vi "Add Command.vi"(8 "error in (no error)":errorcluster, 9 "Index":i32=-1 min=-1 step=1, 10 "Write Command":refnum<class "WriteCommand.lvclass">, 11 "Command Director in":refnum<class "CommandDirector.lvclass">) -> (0 "error out":errorcluster, 3 "Command Director out":refnum<class "CommandDirector.lvclass">)   [LabVIEW 2023, in "HAF.lvlib" / "CommandDirector.lvclass"]
doc: "Adds a Command to a given position in the current collection. If Index is not provided, then adds at the end. Collection is zero indexed so passing 0 will insert at the beginning."
uses:
  CommandDirector.lvclass
  WriteCommand/WriteCommand.lvclass
  CommandDirector.lvclass/CommandDirector.ctl
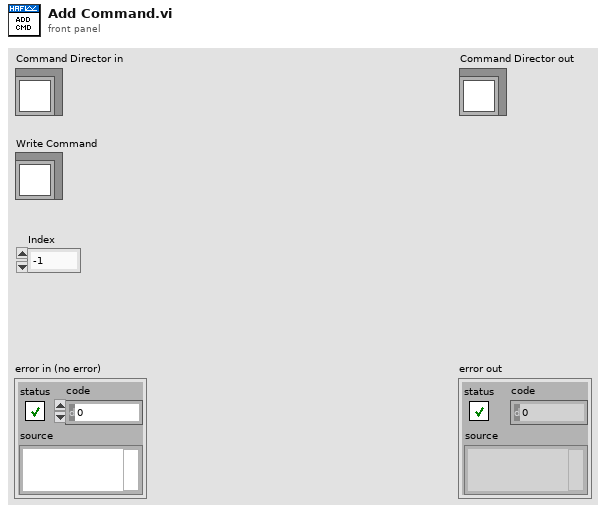
[diagram p1: front panel]
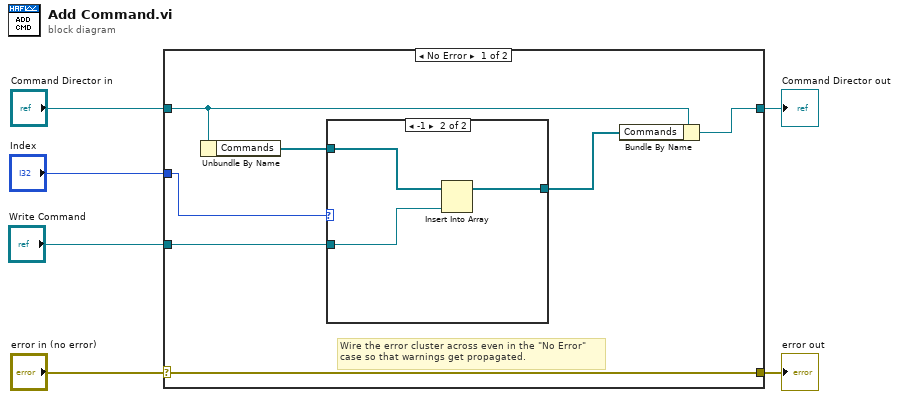
[diagram p0: block diagram]
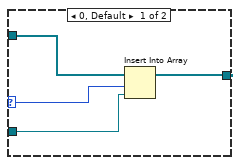
[diagram p2: hidden frame]
diagram:
  n1 = case shown="No Error" "error in (no error)" {
    selector: "error in (no error)" -> [w13 w22]
    tunnel: [w13 w22] -> w5
    tunnel: [w7 w21] -> w3
    tunnel: "Command Director in" -> [w9 w21]
    tunnel: "Index" -> [w11 _]
    tunnel: "Write Command" -> [w10 _]
    frame No Error {
      # "Wire the error cluster across even in the \"No Error\"\ncase so that warnings get propagated."
      n2 = Unbundle By Name(w9) -> ("Commands"=w12:refnum<class "WriteCommand.lvclass">[])
      n3 = case shown="-1" w11 {
        selector: w11 -> [w16 _]
        tunnel: w12 -> [w17 w20]
        tunnel: w10 -> [w15 w19]
        tunnel: [w14 w18] -> w8
        frame 0, Default {
          n4 = Insert Into Array(array=w17, index=w16, new element=w15) -> (w14:refnum<class "WriteCommand.lvclass">[])
        }
        frame -1 {
          n5 = Insert Into Array(array=w20, new element=w19) -> (w18:refnum<class "WriteCommand.lvclass">[])  [unwired: 1 in]
        }
      }
      n6 = Bundle By Name(cluster=w9, "Commands"=w8) -> (w7:refnum<class "CommandDirector.lvclass">)
    }
    frame Error {
    }
  }
  "error out" <- w5
  "Command Director out" <- w3
